vi "SetMenuBar.vi"(8 "error in (no error)":errorcluster, 11 "Gviewer in":refnum<class "Gviewer.lvclass">) -> (0 "error out":errorcluster, 3 "Gviewer out":refnum<class "Gviewer.lvclass">)   [LabVIEW 2020, in "Sgraph_lib_V1.lvlib" / "Gviewer.lvclass"]
doc: "Andre Koelewijn, 3 jan 2021\n\nReplace the panel menu bar by a custom menu bar as defined during initialization"
uses:
  Gviewer.lvclass
  Gviewer.lvclass/Gviewer.ctl
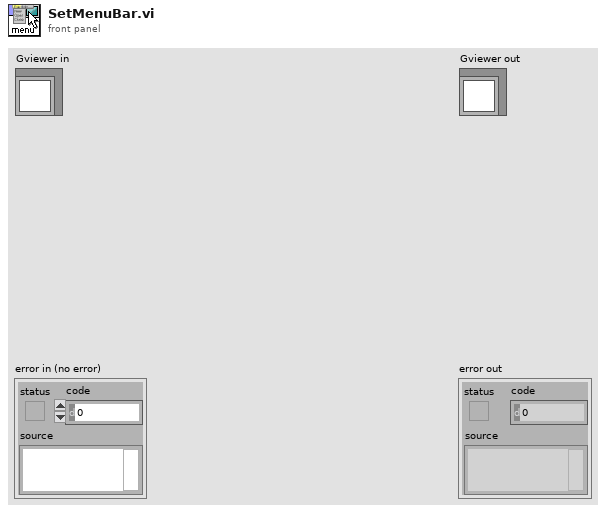
[diagram p1: front panel]
types:
  T1 = typedef "MenuItem.ctl" = cluster{"name":string, "tag":string, "checked":bool, "enabled":bool}
  T2 = typedef "MenuStructure.ctl" = cluster{"After_tag":string, "MenuItems":T1[]}[]
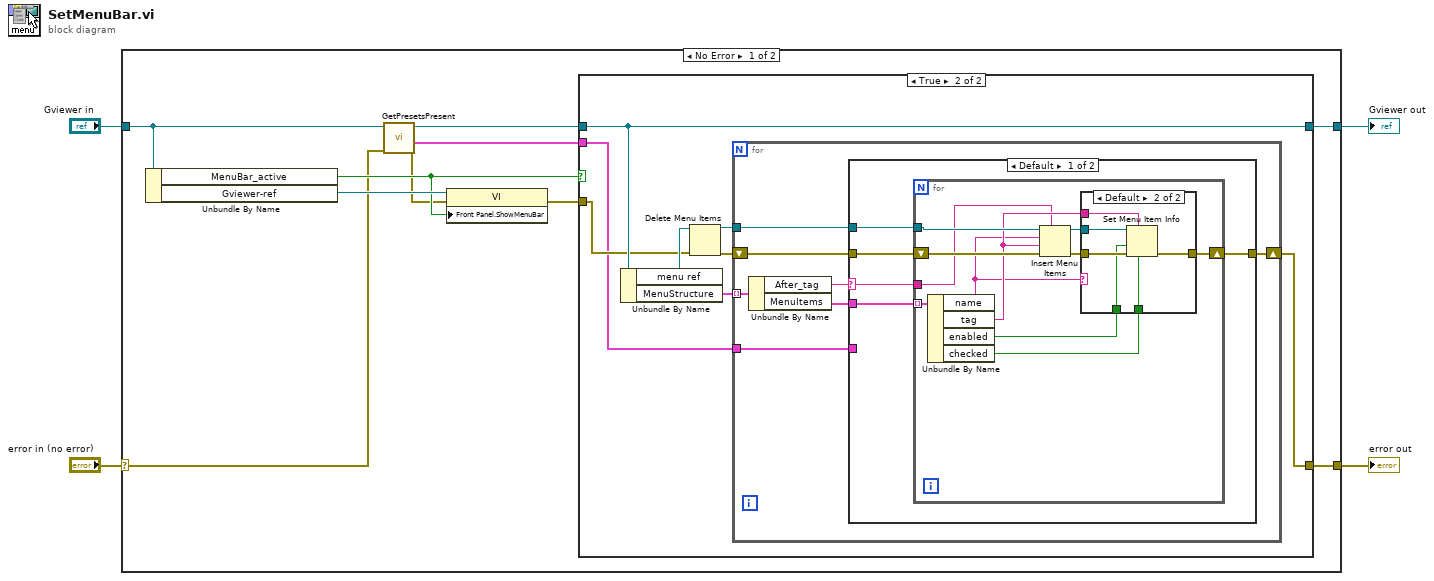
[diagram p0: block diagram]
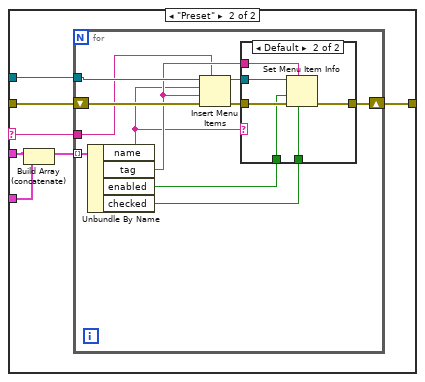
[diagram p4: hidden frame]
diagram:
  n1 = case shown="No Error" "error in (no error)" {
    selector: "error in (no error)" -> [w6 w81]
    tunnel: [w13 w81] -> w3
    tunnel: [w14 w80] -> w1
    tunnel: "Gviewer in" -> [w8 w80]
    frame No Error {
      n2 = Unbundle By Name(w8) -> ("MenuBar_active"=w11:bool, "Gviewer-ref"=w12:refnum<vi>)
      n3 = call "GetPresetsPresent.vi"("error in (no error)"=w6, "Gviewer in"=w8) -> ("error out"=w5:errorcluster, "PresentsInMenu"=w7:T1[], "Gviewer out"=w9:refnum<class "Gviewer.lvclass">)  [unwired: 7 in]
      n4 = property class="VI"(reference=w12, error in=w5, "Front Panel.ShowMenuBar"=w11) -> (error out=w10:errorcluster)  [unwired: 1 out]
      n5 = case shown="True" w11 {
        tunnel: w9 -> [w16 w24]
        tunnel: [w16 w24] -> w14
        tunnel: [w15 w22] -> w13
        tunnel: w10 -> [w15 w19]
        tunnel: w7 -> [_ w17]
        frame False {
        }
        frame True {
          n6 = Unbundle By Name(w24) -> ("menu ref"=w21:refnum<k9>, "MenuStructure"=w23:T2)
          n7 = Delete Menu Items(6:w19, 9:w21) -> (0:w18:errorcluster, 3:w20:refnum<k9>)  [unwired: 2 in]
          n8 = for {
            tunnel: w23 -> [w31] mode=indexing
            shift-right: [w27] -> w22
            shift-left: w18 -> [w28]
            tunnel: w20 -> [w26]
            tunnel: w17 -> [w25]
            n9 = Unbundle By Name(w31) -> ("After_tag"=w29:string, "MenuItems"=w30:T1[])
            n10 = case shown="Default" w29 {
              selector: w29 -> [w35 w61]
              tunnel: w30 -> [w36 w56]
              tunnel: w28 -> [w34 w60]
              tunnel: [w33 w59] -> w27
              tunnel: w26 -> [w32 w58]
              tunnel: w25 -> [_ w57]
              frame Default {
                n11 = for {
                  tunnel: w36 -> [w44] mode=indexing
                  tunnel: w35 -> [w38]
                  shift-right: [w45] -> w33
                  shift-left: w34 -> [w47]
                  tunnel: w32 -> [w43]
                  n12 = Unbundle By Name(w44) -> ("name"=w37:string, "tag"=w39:string, "enabled"=w40:bool, "checked"=w41:bool)
                  n13 = Insert Menu Items(5:w38, 6:w47, 7:w39, 8:w37, 9:w43) -> (0:w46:errorcluster, 3:w42:refnum<k9>)  [unwired: 1 in, 1 out]
                  n14 = case shown="Default" w37 {
                    tunnel: w46 -> [w48 w54]
                    tunnel: [w48 w53] -> w45
                    tunnel: w42 -> [_ w52]
                    tunnel: w41 -> [_ w51]
                    tunnel: w40 -> [_ w50]
                    tunnel: w39 -> [_ w49]
                    frame "app_separator" {
                    }
                    frame Default {
                      n15 = Set Menu Item Info(6:w51, 7:w49, 8:w54, 9:w50, 11:w52) -> (0:w53:errorcluster)  [unwired: 2 in, 1 out]
                    }
                  }
                }
              }
              frame "Preset" {
                n16 = Build Array (concatenate)(w56, w57) -> (w55:T1[])
                n17 = for {
                  tunnel: w55 -> [w69] mode=indexing
                  tunnel: w61 -> [w63]
                  shift-right: [w70] -> w59
                  shift-left: w60 -> [w72]
                  tunnel: w58 -> [w68]
                  n18 = Unbundle By Name(w69) -> ("name"=w62:string, "tag"=w64:string, "enabled"=w65:bool, "checked"=w66:bool)
                  n19 = Insert Menu Items(5:w63, 6:w72, 7:w64, 8:w62, 9:w68) -> (0:w71:errorcluster, 3:w67:refnum<k9>)  [unwired: 1 in, 1 out]
                  n20 = case shown="Default" w62 {
                    tunnel: w71 -> [w73 w79]
                    tunnel: [w73 w78] -> w70
                    tunnel: w67 -> [_ w77]
                    tunnel: w66 -> [_ w76]
                    tunnel: w65 -> [_ w75]
                    tunnel: w64 -> [_ w74]
                    frame "app_separator" {
                    }
                    frame Default {
                      n21 = Set Menu Item Info(6:w76, 7:w74, 8:w79, 9:w75, 11:w77) -> (0:w78:errorcluster)  [unwired: 2 in, 1 out]
                    }
                  }
                }
              }
            }
          }
        }
      }
    }
    frame Error {
    }
  }
  "error out" <- w3
  "Gviewer out" <- w1
